vi "Get Annotation Shown.vi"(8 "error in (no error)":errorcluster, 11 "FSM.Edge in":refnum<class "FSM.Edge.lvclass">) -> (0 "error out":errorcluster, 1 "shown":bool, 3 "FSM.Edge out":refnum<class "FSM.Edge.lvclass">)   [LabVIEW 2015, in "FSM.Edge.lvclass"]
uses:
  FSM.Edge.lvclass
  FSM.Edge.lvclass/FSM.Edge.ctl
  FSM.Annotation/FSM.Annotation.lvclass/FSM.Annotation.ctl
  FSM.Annotation/Read Show.vi
  FSM.Annotation/FSM.Annotation.lvclass
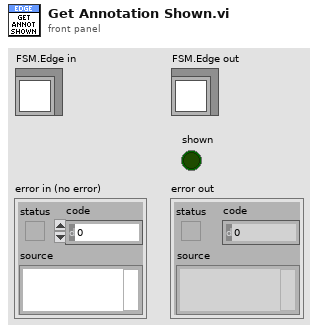
[diagram p1: front panel]
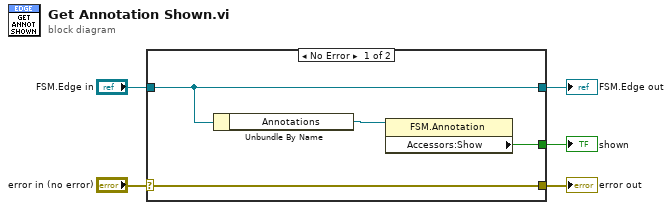
[diagram p0: block diagram]
diagram:
  n1 = case shown="No Error" "error in (no error)" {
    selector: "error in (no error)" -> [w9 w11]
    tunnel: [w9 w11] -> w4
    tunnel: [w8 w10] -> w2
    tunnel: "FSM.Edge in" -> [w8 w10]
    tunnel: [w6 _] -> w1
    frame No Error {
      n2 = Unbundle By Name(w8) -> ("Annotations"=w7:refnum<class "FSM.Annotation.lvclass">)
      n3 = property class="FSM.Annotation"(reference=w7) -> ("Accessors:Show"=w6:bool)  [unwired: 1 in, 2 out]
    }
    frame Error {
    }
  }
  "error out" <- w4
  "FSM.Edge out" <- w2
  "shown" <- w1
